vi "Reference Array to Spreadsheet String.vi"(11 "Control Refs":refnum<vi>[](array[refnum])) -> ()   [LabVIEW 2017]
panel:
  out "error out":errorcluster
  in  "error in (no error)":errorcluster
  in  "format string":string="Test Details: %s\\nDate: %s\nSelected Test: %s\n\nData Snapshot: %s\nTime: %s\nSet Points:\nResistance: %s, RPM: %s, Load Bank: %s\nMeasurments:\nTorque (in*lb),RPM,%s"
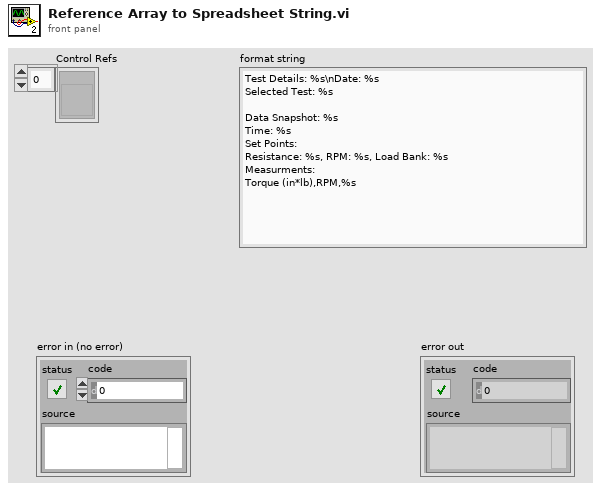
[diagram p1: front panel]
types:
  T1 = typedef "Type Enum.ctl" = enum8{"Void", "I8", "I16", "I32", "I64", "U8", "U16", "U32", "U64", "Single Float", "Double Float", "Extended Float", "Single Complex", "Double Complex", "Extended Complex", "Enum I8 NEVER", "Enum I16 NEVER", "Enum I32 NEVER", "Enum I64 NEVER", "Enum U8", "Enum U16", "Enum U32", "Enum U64", "Single Float With Unit", "Double Float With Unit", "Extended Float With Unit", "Single Complex With Unit", "Double Complex With Unit", "Extended Complex With Unit", "boolU16", "Boolean", "String", "Handle", "Path", "Picture", "C String", "Pascal String", "Tag", "SubString", "Array", "SubArray", "Cluster", "Numeric Cluster", "Variant", "LV Variant", "Measure Data (waveform)", "Refnum", "ExtData", "function", "Typedef", "Poly VI", "bad wire", "LabVIEW Class Instance"}
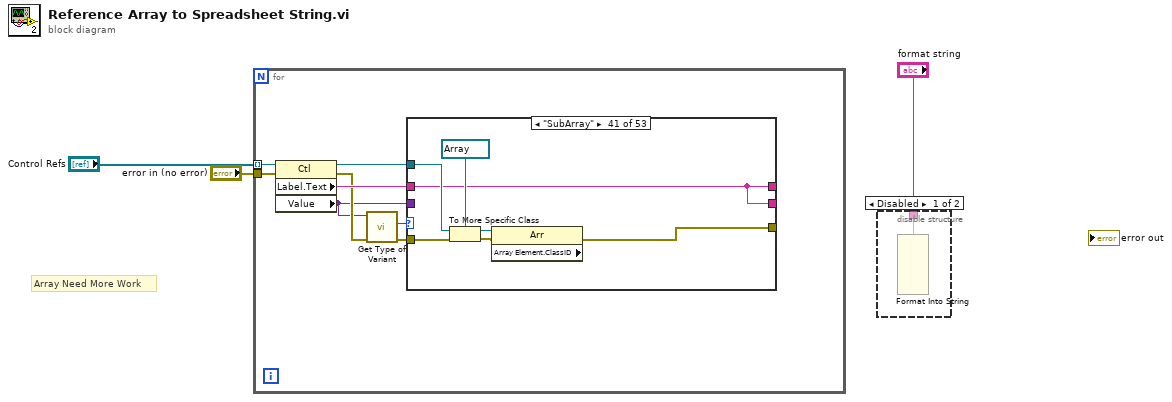
[diagram p0: block diagram]
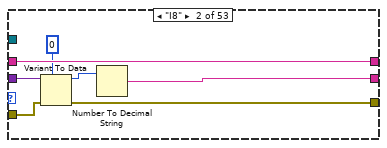
[diagram p4: hidden frame]
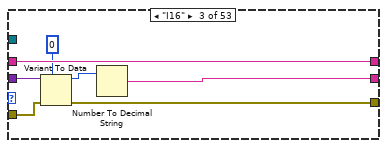
[diagram p5: hidden frame]
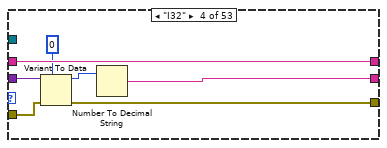
[diagram p6: hidden frame]
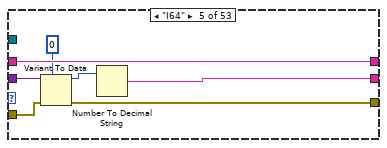
[diagram p7: hidden frame]
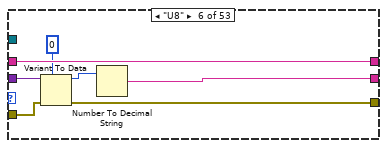
[diagram p8: hidden frame]
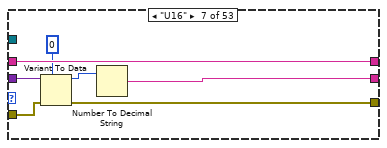
[diagram p9: hidden frame]
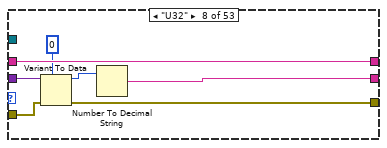
[diagram p10: hidden frame]
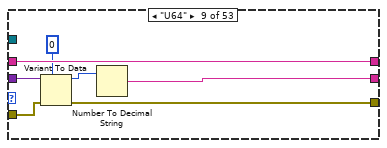
[diagram p11: hidden frame]
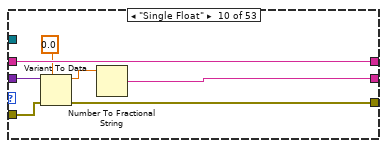
[diagram p12: hidden frame]
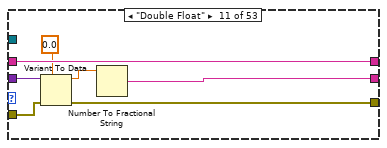
[diagram p13: hidden frame]
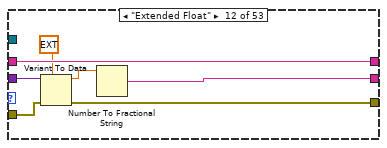
[diagram p14: hidden frame]
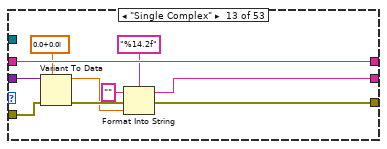
[diagram p15: hidden frame]
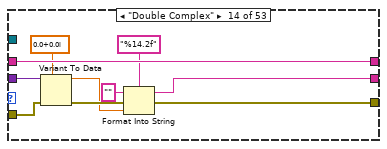
[diagram p16: hidden frame]
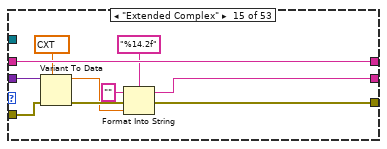
[diagram p17: hidden frame]
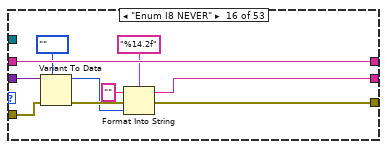
[diagram p18: hidden frame]
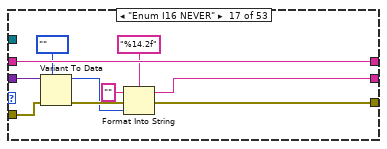
[diagram p19: hidden frame]
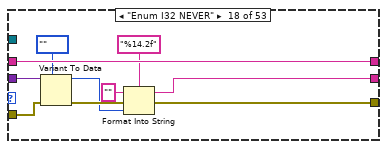
[diagram p20: hidden frame]
diagram:
  # "Array Need More Work"
  n1 = for {
    tunnel: "Control Refs" -> [w10] mode=indexing
    tunnel: "error in (no error)" -> [w7]
    n2 = property class="Ctl"(reference=w10, error in=w7) -> (reference out=w4:refnum<vi>, error out=w8:errorcluster, "Label.Text"=w9:string, "Value"=w6:variant)
    n3 = call <vilib>:"Get Type of Variant.vi"("error in (no error)"=w8, "Data In"=w6) -> ("error out"=w5:errorcluster, "Type Enum"=w11:T1)  [unwired: 8 in]
    n4 = case shown="\"SubArray\"" w11 {
      selector: w11 -> [_ _ _ _ _ _ _ _ _ _ _ _ _ _ _ _ _ _ _ _ _ _ _ _ _ _ _ _ _ _ _ _ w276 _ w290 _ _ _ _ _ _ _ _ _ _ _ _ _ _ _ _ _ _]
      tunnel: w9 -> [w13 w18 w25 w32 w39 w46 w53 w60 w67 w74 w81 w88 w98 w108 w118 w128 w138 w148 w158 w168 w178 w188 w198 w205 w212 w219 w229 w239 w249 w258 w267 w270 w279 w285 w294 w298 w303 w308 w313 w317 w324 _ _ _ _ _ _ _ _ _ _ _ _]
      tunnel: [w13 w18 w25 w32 w39 w46 w53 w60 w67 w74 w81 w88 w98 w108 w118 w128 w138 w148 w158 w168 w178 w188 w198 w205 w212 w219 w229 w239 w249 w258 w267 w270 w279 w285 w294 w298 w303 w308 w313 w317 w324 _ _ _ _ _ _ _ _ _ _ _ _] -> _
      tunnel: [w13 w14 w21 w28 w35 w42 w49 w56 w63 w70 w77 w84 w94 w104 w114 w124 w134 w144 w154 w164 w174 w184 w194 w201 w208 w215 w222 w232 w242 w252 w261 w271 w275 w282 w289 w297 w302 w307 w312 w317 w324 _ _ _ _ _ _ _ _ _ _ _ _] -> _
      tunnel: w6 -> [_ w20 w27 w34 w41 w48 w55 w62 w69 w76 w83 w90 w100 w110 w120 w130 w140 w150 w160 w170 w180 w190 w200 w207 w214 w221 w231 w241 w251 w260 w269 w274 w281 w288 w296 w301 w306 w311 w316 _ _ _ _ _ _ _ _ _ _ _ _ _ _]
      tunnel: w5 -> [w12 w19 w26 w33 w40 w47 w54 w61 w68 w75 w82 w89 w99 w109 w119 w129 w139 w149 w159 w169 w179 w189 w199 w206 w213 w220 w230 w240 w250 w259 w268 w273 w280 w287 w295 w300 w305 w310 w315 w321 w328 _ _ _ _ _ _ _ _ _ _ _ _]
      tunnel: [w12 w17 w24 w31 w38 w45 w52 w59 w66 w73 w80 w87 w95 w105 w115 w125 w135 w145 w155 w165 w175 w185 w195 w203 w210 w217 w226 w236 w246 w255 w264 w272 w277 w286 w291 w299 w304 w309 w314 w318 w325 _ _ _ _ _ _ _ _ _ _ _ _] -> _
      tunnel: w4 -> [_ _ _ _ _ _ _ _ _ _ _ _ _ _ _ _ _ _ _ _ _ _ _ _ _ _ _ _ _ _ _ _ _ _ _ _ _ _ _ w323 w330 _ _ _ _ _ _ _ _ _ _ _ _]
      frame "Void", Default {
      }
      frame "I8" {
        n5 = Variant To Data(error in=w19, type=0, Variant=w20) -> (data=w15:i32, error out=w17:errorcluster)
        n6 = Number To Decimal String(number=w15) -> (decimal integer string=w14:string)  [unwired: 1 in]
      }
      frame "I16" {
        n7 = Variant To Data(error in=w26, type=i16 0, Variant=w27) -> (data=w22:i16, error out=w24:errorcluster)
        n8 = Number To Decimal String(number=w22) -> (decimal integer string=w21:string)  [unwired: 1 in]
      }
      frame "I32" {
        n9 = Variant To Data(error in=w33, type=0, Variant=w34) -> (data=w29:i32, error out=w31:errorcluster)
        n10 = Number To Decimal String(number=w29) -> (decimal integer string=w28:string)  [unwired: 1 in]
      }
      frame "I64" {
        n11 = Variant To Data(error in=w40, type=i64 0, Variant=w41) -> (data=w36:i64, error out=w38:errorcluster)
        n12 = Number To Decimal String(number=w36) -> (decimal integer string=w35:string)  [unwired: 1 in]
      }
      frame "U8" {
        n13 = Variant To Data(error in=w47, type=u8 0, Variant=w48) -> (data=w43:u8, error out=w45:errorcluster)
        n14 = Number To Decimal String(number=w43) -> (decimal integer string=w42:string)  [unwired: 1 in]
      }
      frame "U16" {
        n15 = Variant To Data(error in=w54, type=u16 0, Variant=w55) -> (data=w50:u16, error out=w52:errorcluster)
        n16 = Number To Decimal String(number=w50) -> (decimal integer string=w49:string)  [unwired: 1 in]
      }
      frame "U32" {
        n17 = Variant To Data(error in=w61, type=u32 0, Variant=w62) -> (data=w57:u32, error out=w59:errorcluster)
        n18 = Number To Decimal String(number=w57) -> (decimal integer string=w56:string)  [unwired: 1 in]
      }
      frame "U64" {
        n19 = Variant To Data(error in=w68, type=u64 0, Variant=w69) -> (data=w64:u64, error out=w66:errorcluster)
        n20 = Number To Decimal String(number=w64) -> (decimal integer string=w63:string)  [unwired: 1 in]
      }
      frame "Single Float" {
        n21 = Variant To Data(error in=w75, type=sgl 0.0, Variant=w76) -> (data=w71:sgl, error out=w73:errorcluster)
        n22 = Number To Fractional String(number=w71) -> (F-format string=w70:string)  [unwired: 3 in]
      }
      frame "Double Float" {
        n23 = Variant To Data(error in=w82, type=0.0, Variant=w83) -> (data=w78:dbl, error out=w80:errorcluster)
        n24 = Number To Fractional String(number=w78) -> (F-format string=w77:string)  [unwired: 3 in]
      }
      frame "Extended Float" {
        n25 = Variant To Data(error in=w89, type=ext 0.0, Variant=w90) -> (data=w85:ext, error out=w87:errorcluster)
        n26 = Number To Fractional String(number=w85) -> (F-format string=w84:string)  [unwired: 3 in]
      }
      frame "Single Complex" {
        n27 = Variant To Data(error in=w99, type=csg 0.0+0.0i, Variant=w100) -> (data=w93:csg, error out=w96:errorcluster)
        n28 = Format Into String(format string="%14.2f", initial string="", error in=w96, w93) -> (resulting string=w94:string, error out=w95:errorcluster)
      }
      frame "Double Complex" {
        n29 = Variant To Data(error in=w109, type=cdb 0.0+0.0i, Variant=w110) -> (data=w103:cdb, error out=w106:errorcluster)
        n30 = Format Into String(format string="%14.2f", initial string="", error in=w106, w103) -> (resulting string=w104:string, error out=w105:errorcluster)
      }
      frame "Extended Complex" {
        n31 = Variant To Data(error in=w119, type=cxt 0.0+0.0i, Variant=w120) -> (data=w113:cxt, error out=w116:errorcluster)
        n32 = Format Into String(format string="%14.2f", initial string="", error in=w116, w113) -> (resulting string=w114:string, error out=w115:errorcluster)
      }
      frame "Enum I8 NEVER" {
        n33 = Variant To Data(error in=w129, type=enum16{""}."", Variant=w130) -> (data=w123:enum16{""}, error out=w126:errorcluster)
        n34 = Format Into String(format string="%14.2f", initial string="", error in=w126, w123) -> (resulting string=w124:string, error out=w125:errorcluster)
      }
      frame "Enum I16 NEVER" {
        n35 = Variant To Data(error in=w139, type=enum16{""}."", Variant=w140) -> (data=w133:enum16{""}, error out=w136:errorcluster)
        n36 = Format Into String(format string="%14.2f", initial string="", error in=w136, w133) -> (resulting string=w134:string, error out=w135:errorcluster)
      }
      frame "Enum I32 NEVER" {
        n37 = Variant To Data(error in=w149, type=enum16{""}."", Variant=w150) -> (data=w143:enum16{""}, error out=w146:errorcluster)
        n38 = Format Into String(format string="%14.2f", initial string="", error in=w146, w143) -> (resulting string=w144:string, error out=w145:errorcluster)
      }
      frame "Enum I64 NEVER" {
        n39 = Variant To Data(error in=w159, type=enum16{""}."", Variant=w160) -> (data=w153:enum16{""}, error out=w156:errorcluster)
        n40 = Format Into String(format string="%14.2f", initial string="", error in=w156, w153) -> (resulting string=w154:string, error out=w155:errorcluster)
      }
      frame "Enum U8" {
        n41 = Variant To Data(error in=w169, type=enum8{""}."", Variant=w170) -> (data=w163:enum8{""}, error out=w166:errorcluster)
        n42 = Format Into String(format string="%14.2f", initial string="", error in=w166, w163) -> (resulting string=w164:string, error out=w165:errorcluster)
      }
      frame "Enum U16" {
        n43 = Variant To Data(error in=w179, type=enum16{""}."", Variant=w180) -> (data=w173:enum16{""}, error out=w176:errorcluster)
        n44 = Format Into String(format string="%14.2f", initial string="", error in=w176, w173) -> (resulting string=w174:string, error out=w175:errorcluster)
      }
      frame "Enum U32" {
        n45 = Variant To Data(error in=w189, type=enum32{""}."", Variant=w190) -> (data=w183:enum32{""}, error out=w186:errorcluster)
        n46 = Format Into String(format string="%14.2f", initial string="", error in=w186, w183) -> (resulting string=w184:string, error out=w185:errorcluster)
      }
      frame "Enum U64" {
        n47 = Variant To Data(error in=w199, type=enum32{""}."", Variant=w200) -> (data=w193:enum32{""}, error out=w196:errorcluster)
        n48 = Format Into String(format string="%14.2f", initial string="", error in=w196, w193) -> (resulting string=w194:string, error out=w195:errorcluster)
      }
      frame "Single Float With Unit" {
        n49 = Variant To Data(error in=w206, type=sgl 0.0, Variant=w207) -> (data=w202:sgl, error out=w203:errorcluster)
        n50 = Number To Fractional String(number=w202) -> (F-format string=w201:string)  [unwired: 3 in]
      }
      frame "Double Float With Unit" {
        n51 = Variant To Data(error in=w213, type=0.0, Variant=w214) -> (data=w209:dbl, error out=w210:errorcluster)
        n52 = Number To Fractional String(number=w209) -> (F-format string=w208:string)  [unwired: 3 in]
      }
      frame "Extended Float With Unit" {
        n53 = Variant To Data(error in=w220, type=ext 0.0, Variant=w221) -> (data=w216:ext, error out=w217:errorcluster)
        n54 = Number To Fractional String(number=w216) -> (F-format string=w215:string)  [unwired: 3 in]
      }
      frame "Single Complex With Unit" {
        n55 = Variant To Data(error in=w230, type=csg 0.0+0.0i, Variant=w231) -> (data=w225:csg, error out=w227:errorcluster)
        n56 = Format Into String(format string="%14.2f ", initial string="", error in=w227, w225) -> (resulting string=w222:string, error out=w226:errorcluster)
      }
      frame "Double Complex With Unit" {
        n57 = Variant To Data(error in=w240, type=cdb 0.0+0.0i, Variant=w241) -> (data=w235:cdb, error out=w237:errorcluster)
        n58 = Format Into String(format string="%14.2f ", initial string="", error in=w237, w235) -> (resulting string=w232:string, error out=w236:errorcluster)
      }
      frame "Extended Complex With Unit" {
        n59 = Variant To Data(error in=w250, type=cxt 0.0+0.0i, Variant=w251) -> (data=w245:cxt, error out=w247:errorcluster)
        n60 = Format Into String(format string="%14.2f ", initial string="", error in=w247, w245) -> (resulting string=w242:string, error out=w246:errorcluster)
      }
      frame "boolU16" {
        n61 = Variant To Data(error in=w259, type=FALSE, Variant=w260) -> (data=w254:bool, error out=w256:errorcluster)
        n62 = Format Into String(initial string="", error in=w256, w254) -> (resulting string=w252:string, error out=w255:errorcluster)  [unwired: 1 in]
      }
      frame "Boolean" {
        n63 = Variant To Data(error in=w268, type=FALSE, Variant=w269) -> (data=w263:bool, error out=w265:errorcluster)
        n64 = Format Into String(initial string="", error in=w265, w263) -> (resulting string=w261:string, error out=w264:errorcluster)  [unwired: 1 in]
      }
      frame "String" {
        n65 = Variant To Data(error in=w273, type=w270, Variant=w274) -> (data=w271:string, error out=w272:errorcluster)
      }
      frame "Handle" {
        n66 = Variant To Data(error in=w280, type=w279, Variant=w281) -> (error out=w278:errorcluster)  [unwired: 1 out]
        n67 = Format Into String(error in=w278, w276) -> (resulting string=w275:string, error out=w277:errorcluster)  [unwired: 2 in]
      }
      frame "Path" {
        n68 = Variant To Data(error in=w287, type=path "", Variant=w288) -> (data=w283:path, error out=w286:errorcluster)
        n69 = Path To String(path=w283) -> (string=w282:string)
      }
      frame "Picture" {
        n70 = call "Empty Picture"() -> ("empty picture"=w293:picture)
        n71 = Variant To Data(error in=w295, type=w293, Variant=w296) -> (error out=w292:errorcluster)  [unwired: 1 out]
        n72 = Format Into String(error in=w292, w290) -> (resulting string=w289:string, error out=w291:errorcluster)  [unwired: 2 in]
      }
      frame "C String" {
        n73 = Variant To Data(error in=w300, type=w298, Variant=w301) -> (data=w297:string, error out=w299:errorcluster)
      }
      frame "Pascal String" {
        n74 = Variant To Data(error in=w305, type=w303, Variant=w306) -> (data=w302:string, error out=w304:errorcluster)
      }
      frame "Tag" {
        n75 = Variant To Data(error in=w310, type=w308, Variant=w311) -> (data=w307:string, error out=w309:errorcluster)
      }
      frame "SubString" {
        n76 = Variant To Data(error in=w315, type=w313, Variant=w316) -> (data=w312:string, error out=w314:errorcluster)
      }
      frame "Array" {
        n77 = To More Specific Class(target class=refnum<vi> refnum ("Control Refs"), reference=w323, error in=w321) -> (specific class reference=w322:refnum<vi>, error out=w320:errorcluster)
        n78 = property class="Arr" props=["Array Element", "ClassID"](reference=w322, error in=w320) -> (error out=w318:errorcluster)  [unwired: 2 out]
      }
      frame "SubArray" {
        n79 = To More Specific Class(target class=refnum<vi> refnum ("Control Refs"), reference=w330, error in=w328) -> (specific class reference=w329:refnum<vi>, error out=w327:errorcluster)
        n80 = property class="Arr" props=["Array Element", "ClassID"](reference=w329, error in=w327) -> (error out=w325:errorcluster)  [unwired: 2 out]
      }
      frame "Cluster" {
      }
      frame "Numeric Cluster" {
      }
      frame "Variant" {
      }
      frame "LV Variant" {
      }
      frame "Measure Data (waveform)" {
      }
      frame "Refnum" {
      }
      frame "ExtData" {
      }
      frame "function" {
      }
      frame "Typedef" {
      }
      frame "Poly VI" {
      }
      frame "bad wire" {
      }
      frame "LabVIEW Class Instance" {
      }
    }
  }
  n81 = disable-structure shown="Disabled" {
    disable-tunnel: "format string" -> [w331 _]
    frame Disabled {
      n82 = Format Into String(format string=w331) -> ()  [unwired: 7 in, 2 out]
    }
    frame Enabled {
    }
  }
